vi "ADCP_get_data_packet_parameters_list.vi"(8 "error in (no error)":errorcluster, 10 "Data Packet Name":string, 11 "ADCP In":refnum<class "ADCP.lvclass">) -> (0 "error out":errorcluster, 1 "Parameter names":string[](array[string]), 2 "Parameters":T1(array[cluster]), 3 "ADCP out":refnum<class "ADCP.lvclass">)   [LabVIEW 2017, in "ADCP.lvclass"]
uses:
  ADCP.lvclass
  ADCP.lvclass/ADCP.ctl
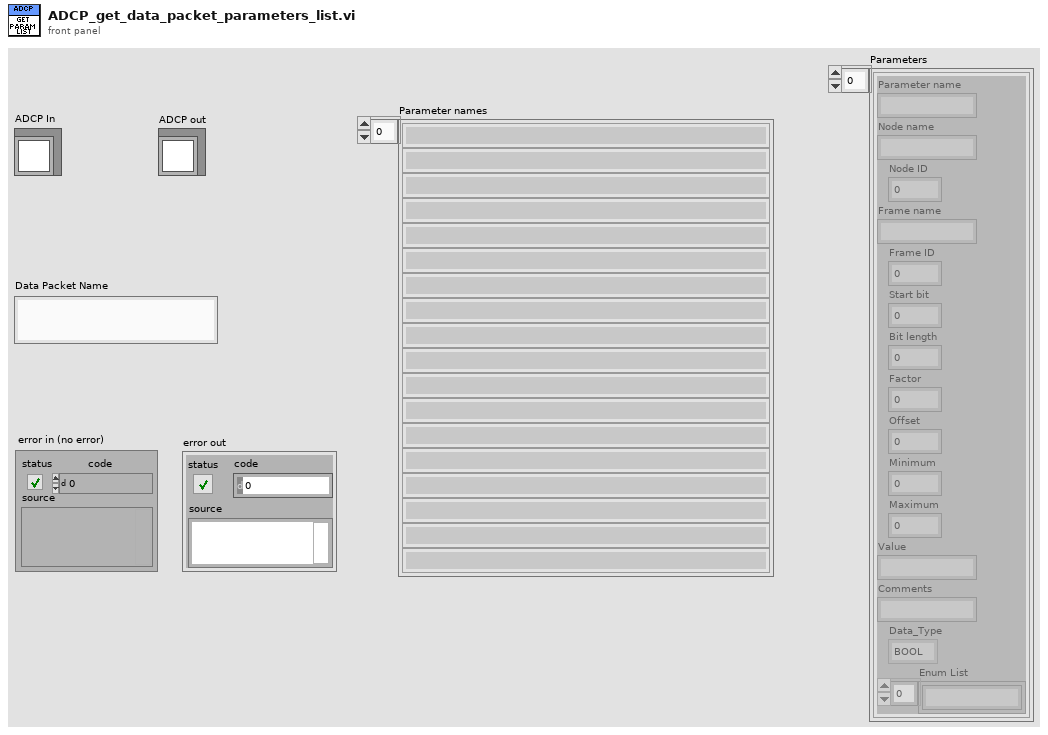
[diagram p1: front panel]
types:
  T1 = cluster{"Parameter name":string, "Node name":string, "Node ID":u8, "Frame name":string, "Frame ID":u8, "Start bit":u32, "Bit length":u32, "Factor":dbl, "Offset":dbl, "Minimum":dbl, "Maximum":dbl, "Value":string, "Comments":string, "Data_Type":enum16{"BOOL", "UNSIGNED", "SIGNED", "FLOAT32", "ENUM"}, "Enum List":string[]}[]
  T2 = typedef "ADCP.lvclass/ADCP_Data_Packet_Transmit_Mode.ctl" = enum16{"Disable", "Single", "Cyclic", "Repeat"}
  T3 = cluster{"Parameters":cluster{"Parameter name":string, "Node name":string, "Node ID":u8, "Frame name":string, "Frame ID":u8, "Start bit":u32, "Bit length":u32, "Factor":dbl, "Offset":dbl, "Minimum":dbl, "Maximum":dbl, "Value":string, "Comments":string, "Data_Type":enum16{"BOOL", "UNSIGNED", "SIGNED", "FLOAT32", "ENUM"}, "Enum List":string[]}[], "Priority":enum16{"LOW", "HIGH"}, "Node name":string, "Node ID":u8, "Frame name":string, "Frame ID":u8, "Data":u32, "Raw bytes":u8[], "Processed bytes":u8[], "Tx count":i32, "Last Tx Time":u32, "Tx interval":u32, "Rx count":i32, "Last Rx Time":u32, "Rx interval":u32, "Tx Enable":bool, "Tx mode":T2, "Repeat/Cyclic Tx interval":u32, "Repeat count":u16}[]
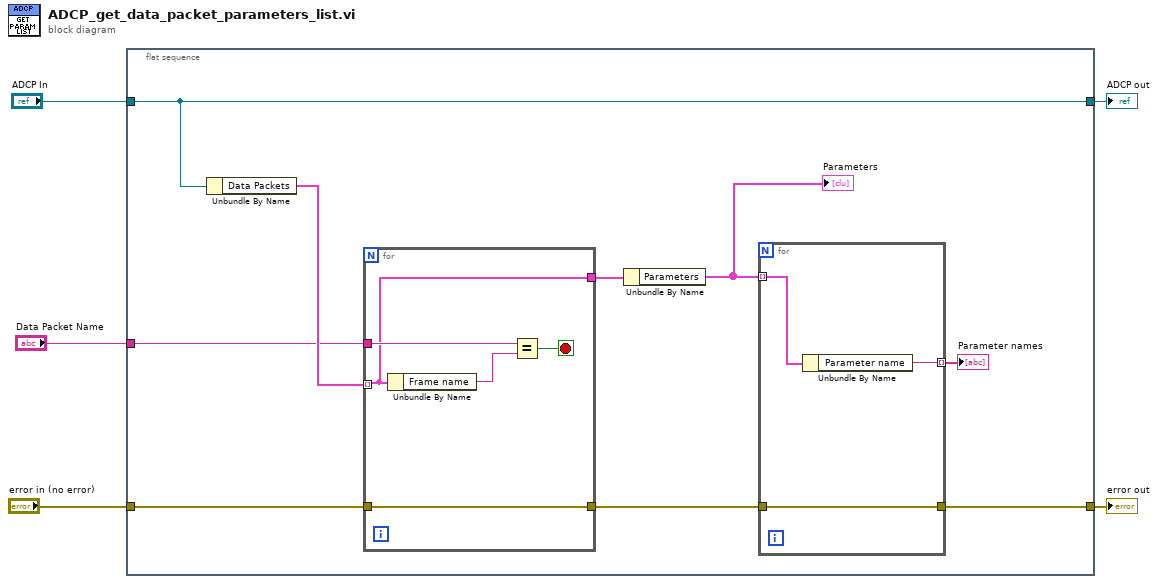
[diagram p0: block diagram]
diagram:
  n1 = flat-sequence {
    tunnel: "ADCP In" -> [w6]
    tunnel: "error in (no error)" -> [w14]
    tunnel: "Data Packet Name" -> [w12]
    tunnel: [w9] -> w2
    tunnel: [w6] -> w1
    frame #0 {
      n2 = Unbundle By Name(w6) -> ("Data Packets"=w13:T3)
      n3 = for {
        tunnel: w14 -> [w20]
        tunnel: w13 -> [w18] mode=indexing
        tunnel: w12 -> [w21]
        tunnel: [w20] -> w10
        tunnel: [w18] -> w11
        stop <- w19 stop-if-true
        n4 = Unbundle By Name(w18) -> ("Frame name"=w22:string)
        n5 = Equal?(x=w21, y=w22) -> (x = y?=w19:bool)
      }
      n6 = Unbundle By Name(w11) -> ("Parameters"=w8:T1)
      "Parameters" <- w8
      n7 = for {
        tunnel: w10 -> [w17]
        tunnel: [w17] -> w9
        tunnel: w8 -> [w16] mode=indexing
        tunnel: [w15] -> w7 mode=indexing
        n8 = Unbundle By Name(w16) -> ("Parameter name"=w15:string)
      }
      "Parameter names" <- w7
    }
  }
  "error out" <- w2
  "ADCP out" <- w1
